vi "Binary Search Sorted Array.vi"(10 "Element":u32, 11 "Sorted Array":u32[](array[numeric])) -> (2 "Found?":bool)   [LabVIEW 2020]
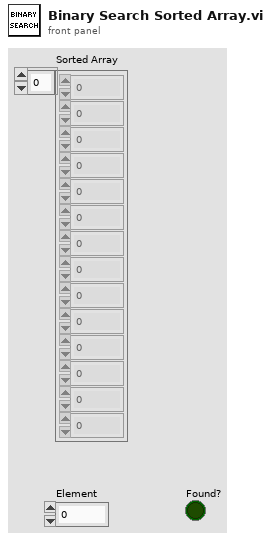
[diagram p1: front panel]
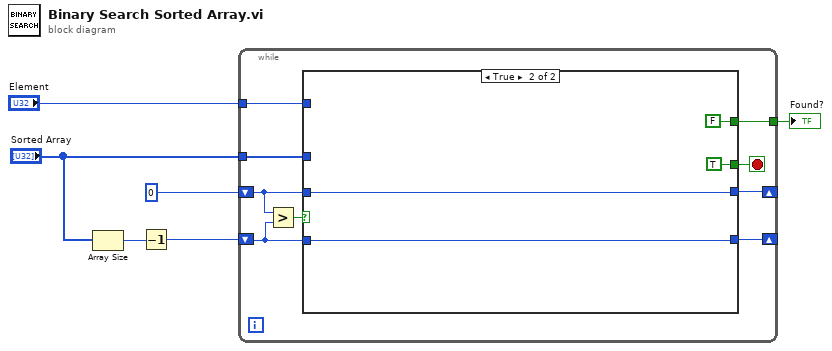
[diagram p0: block diagram]
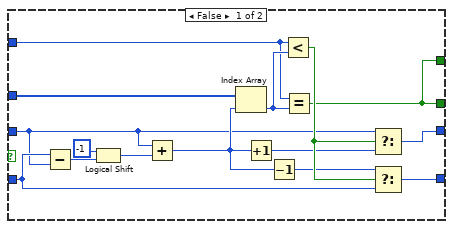
[diagram p2: hidden frame]
diagram:
  n1 = Array Size(array="Sorted Array") -> (size(s)=w6:i32)
  n2 = Decrement(x=w6) -> (x-1=w5:i32)
  n3 = while {
    shift-right: [w10] -> _
    shift-left: w5 -> [w14]
    shift-right: [w9] -> _
    shift-left: 0 -> [w15]
    tunnel: "Sorted Array" -> [w12]
    tunnel: "Element" -> [w11]
    tunnel: [w7] -> w1
    stop <- w8 stop-if-true
    n4 = Greater?(x=w15, y=w14) -> (0:w13:bool)
    n5 = case shown="True" w13 {
      tunnel: w15 -> [w18 w32]
      tunnel: w14 -> [w28 w33]
      tunnel: w12 -> [w29 _]
      tunnel: w11 -> [w23 _]
      tunnel: [w27 w33] -> w10
      tunnel: [w26 w32] -> w9
      tunnel: [w21 TRUE] -> w8
      tunnel: [w21 FALSE] -> w7
      frame False {
        n6 = Subtract(x=w28, y=w18) -> (x-y=w20:i32)
        n7 = Logical Shift(y=i16 -1, x=w20) -> (x << y=w22:i32)
        n8 = Add(x=w18, y=w22) -> (x+y=w19:i32)
        n9 = Index Array(array=w29, index=w19) -> (element=w24:u32)
        n10 = Increment(x=w19) -> (x+1=w17:i32)
        n11 = Decrement(x=w19) -> (x-1=w16:i32)
        n12 = Less?(x=w23, y=w24) -> (x < y?=w25:bool)
        n13 = Equal?(x=w23, y=w24) -> (x = y?=w21:bool)
        n14 = Select(t=w18, s=w25, f=w17) -> (s? t:f=w26:i32)
        n15 = Select(t=w16, s=w25, f=w28) -> (s? t:f=w27:i32)
      }
      frame True {
      }
    }
  }
  "Found?" <- w1
